vi "Server.vi"() -> ()   [LabVIEW 2019]
panel:
  out "Table":string[][](table)
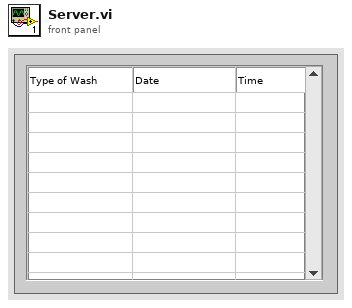
[diagram p1: front panel]
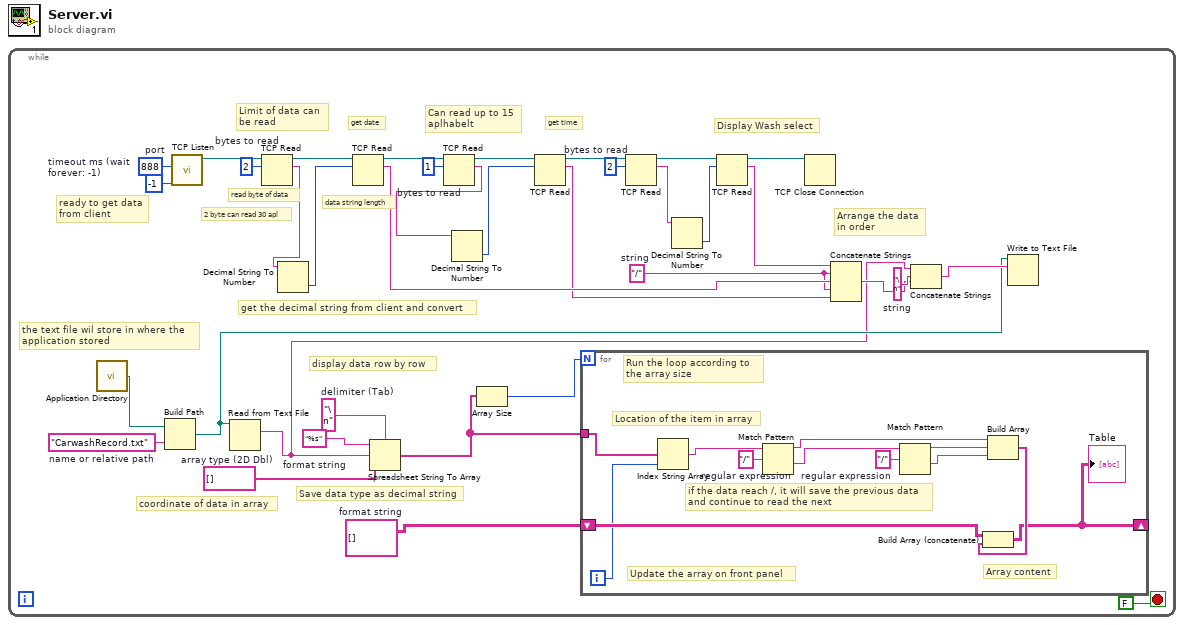
[diagram p0: block diagram]
diagram:
  n1 = while {
    stop <- FALSE stop-if-true
    w6 = "CarwashRecord.txt"  # name or relative path
    w7 = string[][] []  # format string
    w10 = string[] []  # array type (2D Dbl)
    w11 = "%s"  # format string
    w12 = "\n"  # delimiter (Tab)
    w17 = "\n"  # string
    w1 = "/"  # string
    w24 = 2  # bytes to read
    w25 = 1  # bytes to read
    w26 = 2  # bytes to read
    w35 = -1  # timeout ms (wait forever: -1)
    w36 = u16 888  # port
    # "Arrange the data\nin order"
    # "ready to get data\nfrom client"
    # "coordinate of data in array"
    # "Save data type as decimal string"
    # "display data row by row"
    # "the text file wil store in where the \napplication stored"
    # "Can read up to 15\naplhabelt"
    # "Limit of data can \nbe read"
    # "data string length"
    # "get the decimal string from client and convert"
    # "2 byte can read 30 apl"
    # "read byte of data"
    # "Display Wash select"
    # "get time"
    # "get date"
    n2 = call <vilib>:"Application Directory.vi"() -> ("Application Directory"=w8:path)
    n3 = Build Path(base path=w8, name or relative path=w6) -> (appended path=w13:path)
    n4 = call <vilib>:"TCP Listen.vi"("timeout ms (wait forever: -1)"=w35, "port"=w36) -> ("connection ID"=w34:refnum<k5>)  [unwired: 5 in, 4 out]
    n5 = Read from Text File(file (use dialog)=w13) -> (text=w4:string)  [unwired: 3 in, 3 out]
    n6 = TCP Read(connection ID=w34, bytes to read=w26) -> (connection ID out=w33:refnum<k5>, data out=w28:string)  [unwired: 3 in, 1 out]
    n7 = Decimal String To Number(string=w28) -> (number=w27:i32)  [unwired: 2 in, 1 out]
    n8 = TCP Read(connection ID=w33, bytes to read=w27) -> (connection ID out=w32:refnum<k5>, data out=w15:string)  [unwired: 3 in, 1 out]
    n9 = Spreadsheet String To Array(delimiter (Tab)=w12, format string=w11, spreadsheet string=w4, array type (2D Dbl)=w10) -> (array=w5:string[])
    n10 = TCP Read(connection ID=w32, bytes to read=w25) -> (connection ID out=w31:refnum<k5>, data out=w23:string)  [unwired: 3 in, 1 out]
    n11 = Decimal String To Number(string=w23) -> (number=w22:i32)  [unwired: 2 in, 1 out]
    n12 = Array Size(array=w5) -> (size(s)=w9:i32)
    n13 = TCP Read(connection ID=w31, bytes to read=w22) -> (connection ID out=w30:refnum<k5>, data out=w2:string)  [unwired: 3 in, 1 out]
    n14 = for {
      N: w9 -> [_]
      shift-right: [w38] -> _
      shift-left: w7 -> [w48]
      tunnel: w5 -> [w37]
      i -> [w47]
      w42 = "/"  # regular expression
      w45 = "/"  # regular expression
      # "Update the array on front panel"
      # "Location of the item in array"
      # "if the data reach /, it will save the previous data\nand continue to read the next"
      # "Array content"
      # "Run the loop according to\nthe array size"
      n15 = Index String Array(1:w47, 2:w37) -> (0:w46:string)  [unwired: 1 in]
      n16 = Match Pattern(string=w46, regular expression=w45) -> (before substring=w44:string, after substring=w43:string)  [unwired: 1 in, 2 out]
      n17 = Match Pattern(string=w43, regular expression=w42) -> (before substring=w41:string, after substring=w40:string)  [unwired: 1 in, 2 out]
      n18 = Build Array "Build Array"(w44, w41, w40) -> (w39:string[])
      n19 = Build Array (concatenate) "Build Array"(w48, w39) -> (w38:string[][])
      "Table" <- w38
    }
    n20 = TCP Read(connection ID=w30, bytes to read=w24) -> (connection ID out=w29:refnum<k5>, data out=w21:string)  [unwired: 3 in, 1 out]
    n21 = Decimal String To Number(string=w21) -> (number=w20:i32)  [unwired: 2 in, 1 out]
    n22 = TCP Read(connection ID=w29, bytes to read=w20) -> (connection ID out=w19:refnum<k5>, data out=w18:string)  [unwired: 3 in, 1 out]
    n23 = TCP Close Connection(connection ID=w19) -> ()  [unwired: 2 in, 2 out]
    n24 = Concatenate Strings "Concatenate Strings"(w18, w1, w15, w1, w2) -> (w14:string)
    n25 = Concatenate Strings "Concatenate Strings"(w4, w17, w14) -> (w16:string)
    n26 = Write to Text File(file (use dialog)=w13, text=w16) -> ()  [unwired: 2 in, 3 out]
  }
